vi "Frekans_Tablo_Doldur.vi"(10 "Table Reference in":refnum<vi>, 11 "appended array in":dbl[][](array[numeric])) -> (1 "Test Result":bool, 2 "Table Values":string[][](array[string]), 3 "appended array Out":dbl[][](array[numeric]))   [LabVIEW 2014]
uses:
  TestStandInteraction/VeriPaylasim_Globali.vi
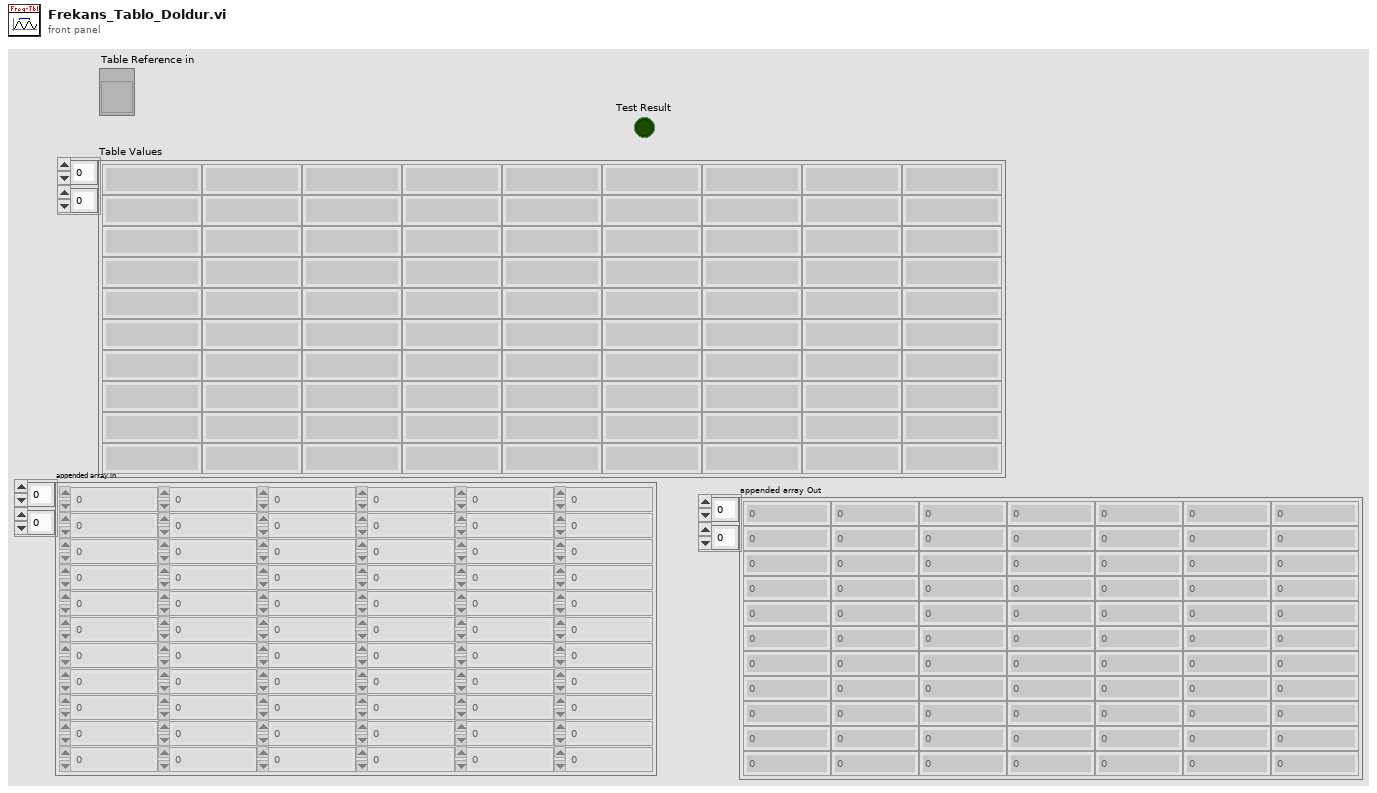
[diagram p1: front panel]
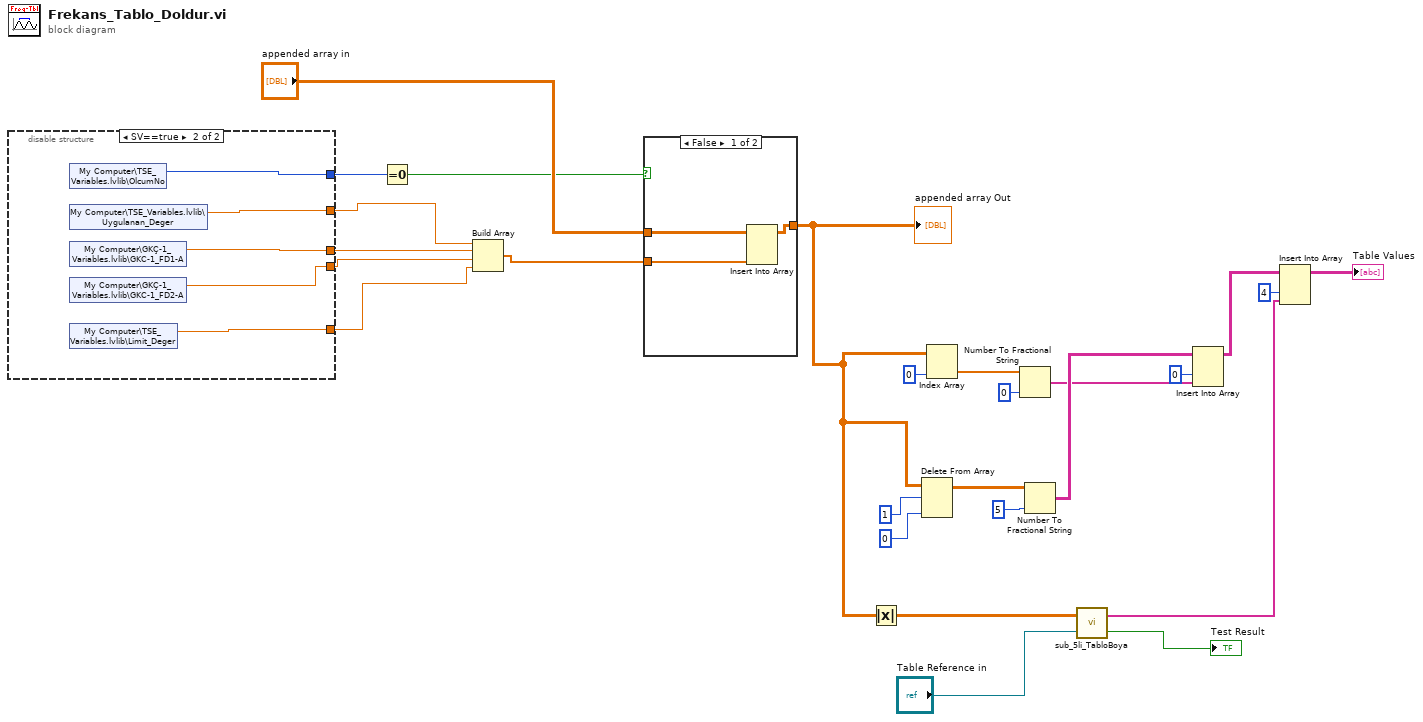
[diagram p0: block diagram]
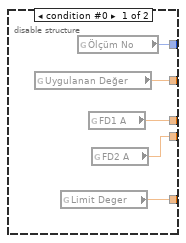
[diagram p2: hidden frame]
diagram:
  n1 = disable-structure shown="SV==true" {
    disable-tunnel: [w31 w32] -> w21
    disable-tunnel: [w30 w34] -> w18
    disable-tunnel: [w29 w36] -> w4
    disable-tunnel: [w28 w35] -> w3
    disable-tunnel: [w27 w33] -> w2
    frame condition #0 {
      n2 = global read "VeriPaylasim_Globali.vi" "Uygulanan Değer"() -> (w31:dbl)
      n3 = global read "VeriPaylasim_Globali.vi" "Limit Deger"() -> (w27:dbl)
      n4 = global read "VeriPaylasim_Globali.vi" "Ölçüm No"() -> (w30:u16)
      n5 = global read "VeriPaylasim_Globali.vi" "FD1 A"() -> (w29:dbl)
      n6 = global read "VeriPaylasim_Globali.vi" "FD2 A"() -> (w28:dbl)
    }
    frame condition #1 (active) {
      n7 = shared-variable "My Computer\\TSE_Variables.lvlib\\OlcumNo"() -> (w34:u16)  [unwired: 1 in, 1 out]
      n8 = shared-variable "My Computer\\TSE_Variables.lvlib\\Uygulanan_Deger"() -> (w32:dbl)  [unwired: 1 in, 1 out]
      n9 = shared-variable "My Computer\\GKÇ-1_Variables.lvlib\\GKC-1_FD1-A"() -> (w36:dbl)  [unwired: 1 in, 1 out]
      n10 = shared-variable "My Computer\\GKÇ-1_Variables.lvlib\\GKC-1_FD2-A"() -> (w35:dbl)  [unwired: 1 in, 1 out]
      n11 = shared-variable "My Computer\\TSE_Variables.lvlib\\Limit_Deger"() -> (w33:dbl)  [unwired: 1 in, 1 out]
    }
  }
  n12 = Equal To 0?(x=w18) -> (x = 0?=w17:bool)
  n13 = Build Array(w21, w4, w3, w2) -> (w20:dbl[])
  n14 = case shown="False" w17 {
    tunnel: w20 -> [w37 _]
    tunnel: [w38 w40] -> w7
    tunnel: "appended array in" -> [w39 w40]
    frame False {
      n15 = Insert Into Array(array=w39, new element=w37) -> (w38:dbl[][])  [unwired: 2 in]
    }
    frame True {
    }
  }
  "appended array Out" <- w7
  n16 = Absolute Value(x=w7) -> (abs(x)=w1:dbl[][])
  n17 = Delete From Array "Delete From Array"(array=w7, length=1, index (col)=0 ("disabled index (col)")) -> (array with subset deleted=w6:dbl[][])  [unwired: 1 in, 1 out]
  n18 = Index Array "Index Array"(array=w7, index (col)=0 ("disabled index (col)")) -> (element=w14:dbl[])  [unwired: 1 in]
  n19 = Number To Fractional String(number=w14, precision (6)=i16 0) -> (F-format string=w10:string[])  [unwired: 2 in]
  n20 = Number To Fractional String(number=w6, precision (6)=i16 5) -> (F-format string=w11:string[][])  [unwired: 2 in]
  n21 = call "sub_5li_TabloBoya.vi"("Table in"="Table Reference in", "Tablo Degerleri"=w1) -> ("Test Result"=→"Test Result":bool, "RESULTS"=w24:string[])
  n22 = Insert Into Array(array=w11, index (col)=0 ("disabled index (col)"), new element=w10) -> (w5:string[][])  [unwired: 1 in]
  n23 = Insert Into Array(array=w5, index (col)=4 ("disabled index (col)"), new element=w24) -> (→"Table Values":string[][])  [unwired: 1 in]
